vi "Encoder.vi"() -> ()   [LabVIEW 2018]
panel:
  out "Counter Value 3":dbl
  in  "Reset3":bool
  out "error out":errorcluster
  out "Counter Value 2":dbl
  out "Counter Value":dbl
  in  "Reset2":bool
  in  "Reset":bool
  in  "stop":bool
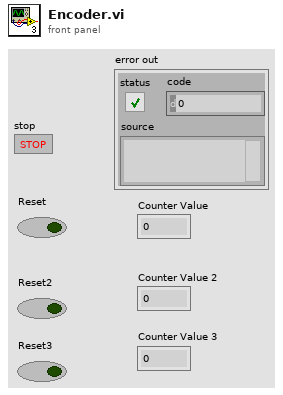
[diagram p1: front panel]
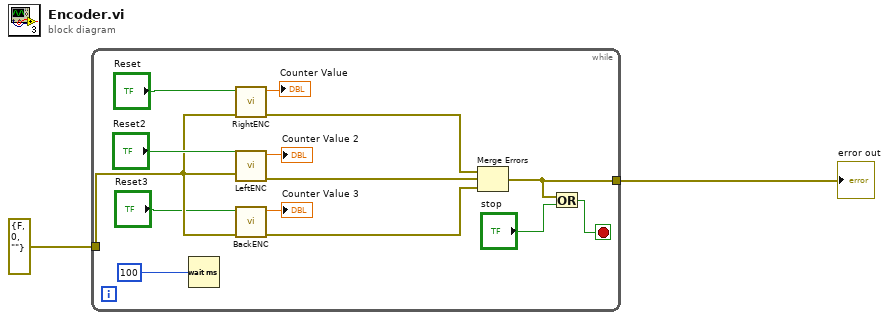
[diagram p0: block diagram]
diagram:
  n1 = while {
    tunnel: errorcluster {FALSE, 0, ""} -> [w6]
    tunnel: [w7] -> w1
    stop <- w8 stop-if-true
    n2 = Wait (ms)(milliseconds to wait=100) -> ()  [unwired: 1 out]
    n3 = call "RightENC.vi"("error in (no error)"=w6, "Reset"="Reset") -> ("error out"=w11:errorcluster, "Counter Value"=→"Counter Value":dbl)  [unwired: 8 in]
    n4 = call "LeftENC.vi"("error in (no error)"=w6, "Reset"="Reset2") -> ("error out"=w10:errorcluster, "Counter Value"=→"Counter Value 2":dbl)  [unwired: 8 in]
    n5 = call "BackENC.vi"("error in (no error)"=w6, "Reset"="Reset3") -> ("error out"=w4:errorcluster, "Counter Value"=→"Counter Value 3":dbl)  [unwired: 8 in]
    n6 = Merge Errors(w11, w10, w4) -> (w7:errorcluster)
    n7 = Or(x=w7, y="stop") -> (x .or. y?=w8:bool)
  }
  "error out" <- w1
